vi "Plot Center of Mass.vi"(0 "Image":T1, 1 "Feature Ponts":cluster{"X":dbl, "Y":dbl}[](array[cluster]), 3 "error in":errorcluster, 4 "Color":u32(colorbox)=65280) -> (7 "Image Out":T1, 10 "error out":errorcluster)   [LabVIEW 2012, in "Visual Analyser.lvlib"]
uses:
  Visual Analyser.lvlib
  <vilib>/vision/Image Controls.llb/IMAQ Image.ctl
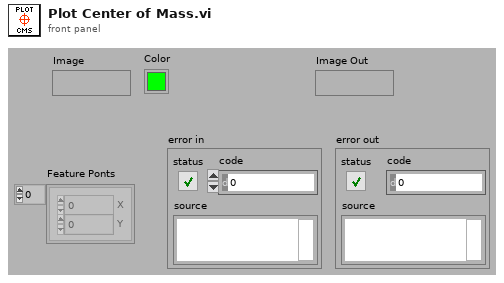
[diagram p1: front panel]
types:
  T1 = typedef "IMAQ Image.ctl" = refnum<image>
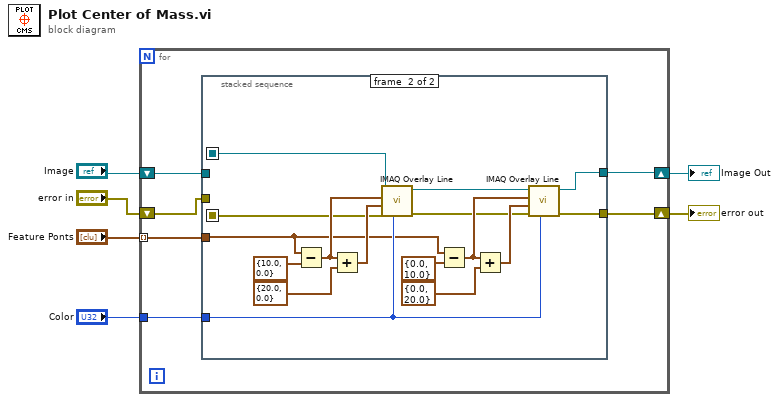
[diagram p0: block diagram]
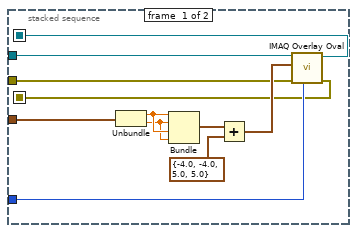
[diagram p2: hidden frame]
diagram:
  n1 = for {
    shift-right: [w10] -> w5
    shift-left: "Image" -> [w12]
    tunnel: "Feature Ponts" -> [w9] mode=indexing
    tunnel: "Color" -> [w11]
    shift-right: [w7] -> w1
    shift-left: "error in" -> [w8]
    n2 = stacked-sequence {
      seq-local: [w22 _] -> [_ w27]
      seq-local: [w14 _] -> [_ w25]
      tunnel: w9 -> [w15 w29]
      tunnel: w12 -> [w23 _]
      tunnel: w11 -> [w21 w31]
      tunnel: [_ w28] -> w10
      tunnel: w8 -> [w13 _]
      tunnel: [_ w24] -> w7
      frame #0 {
        n3 = Unbundle(w15) -> ("X"=w20:dbl, "Y"=w19:dbl)
        n4 = Bundle("X"=w20, "Y"=w19, "X"=w20, "Y"=w19) -> (w18:cluster{"X":dbl, "Y":dbl, "X":dbl, "Y":dbl})  [unwired: 1 out]
        n5 = Add(x=w18, y=cluster{"y":sgl, "x":sgl, "y":sgl, "x":sgl} {"y"=-4.0, "x"=-4.0, "y"=5.0, "x"=5.0}) -> (x+y=w16:cluster{dbl, dbl, dbl, dbl})
        n6 = call "IMAQ Overlay Oval"("Color"=w21, "error in (no error)"=w13, "Bounding Rectangle"=w16, "Image"=w23) -> ("error out"=w14:errorcluster, "Image Out"=w22:T1)  [unwired: 2 in, 4 out]
      }
      frame #1 {
        n7 = Subtract(x=w29, y=cluster{"x":sgl, "y":sgl} {"x"=10.0, "y"=0.0}) -> (x-y=w38:cluster{dbl, dbl})
        n8 = Add(x=w38, y=cluster{"x":sgl, "y":sgl} {"x"=20.0, "y"=0.0}) -> (x+y=w36:cluster{dbl, dbl})
        n9 = call "IMAQ Overlay Line"("Color"=w31, "error in (no error)"=w25, "End Point"=w36, "Start Point"=w38, "Image"=w27) -> ("error out"=w26:errorcluster, "Image Out"=w30:T1)  [unwired: 1 in, 4 out]
        n10 = Subtract(x=w29, y=cluster{"x":sgl, "y":sgl} {"x"=0.0, "y"=10.0}) -> (x-y=w34:cluster{dbl, dbl})
        n11 = Add(x=w34, y=cluster{"x":sgl, "y":sgl} {"x"=0.0, "y"=20.0}) -> (x+y=w35:cluster{dbl, dbl})
        n12 = call "IMAQ Overlay Line"("Color"=w31, "error in (no error)"=w26, "End Point"=w35, "Start Point"=w34, "Image"=w30) -> ("error out"=w24:errorcluster, "Image Out"=w28:T1)  [unwired: 1 in, 4 out]
      }
    }
  }
  "Image Out" <- w5
  "error out" <- w1
